vi "Periodic Tasks.vi"(0 "error in":errorcluster) -> ()   [LabVIEW 2020]
doc: "All TeleOperated, Autonomous, and Test controller logic are located here. Sensor reads and actuator commands are run inside of parallel loops. Most FRC 4265 code should be placed here."
uses:
  dsdata.vi
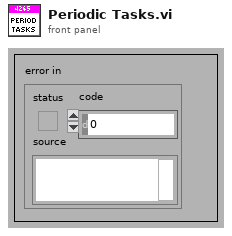
[diagram p1: front panel]
types:
  T1 = typedef "WPI_DriverStationRobotMode2.ctl" = enum16{"Autonomous Disabled", "Autonomous Enabled", "Teleop Disabled", "Teleop Enabled", "Disconnected", "Finish", "Test Disabled", "Test Enabled", "Emergency Stopped"}
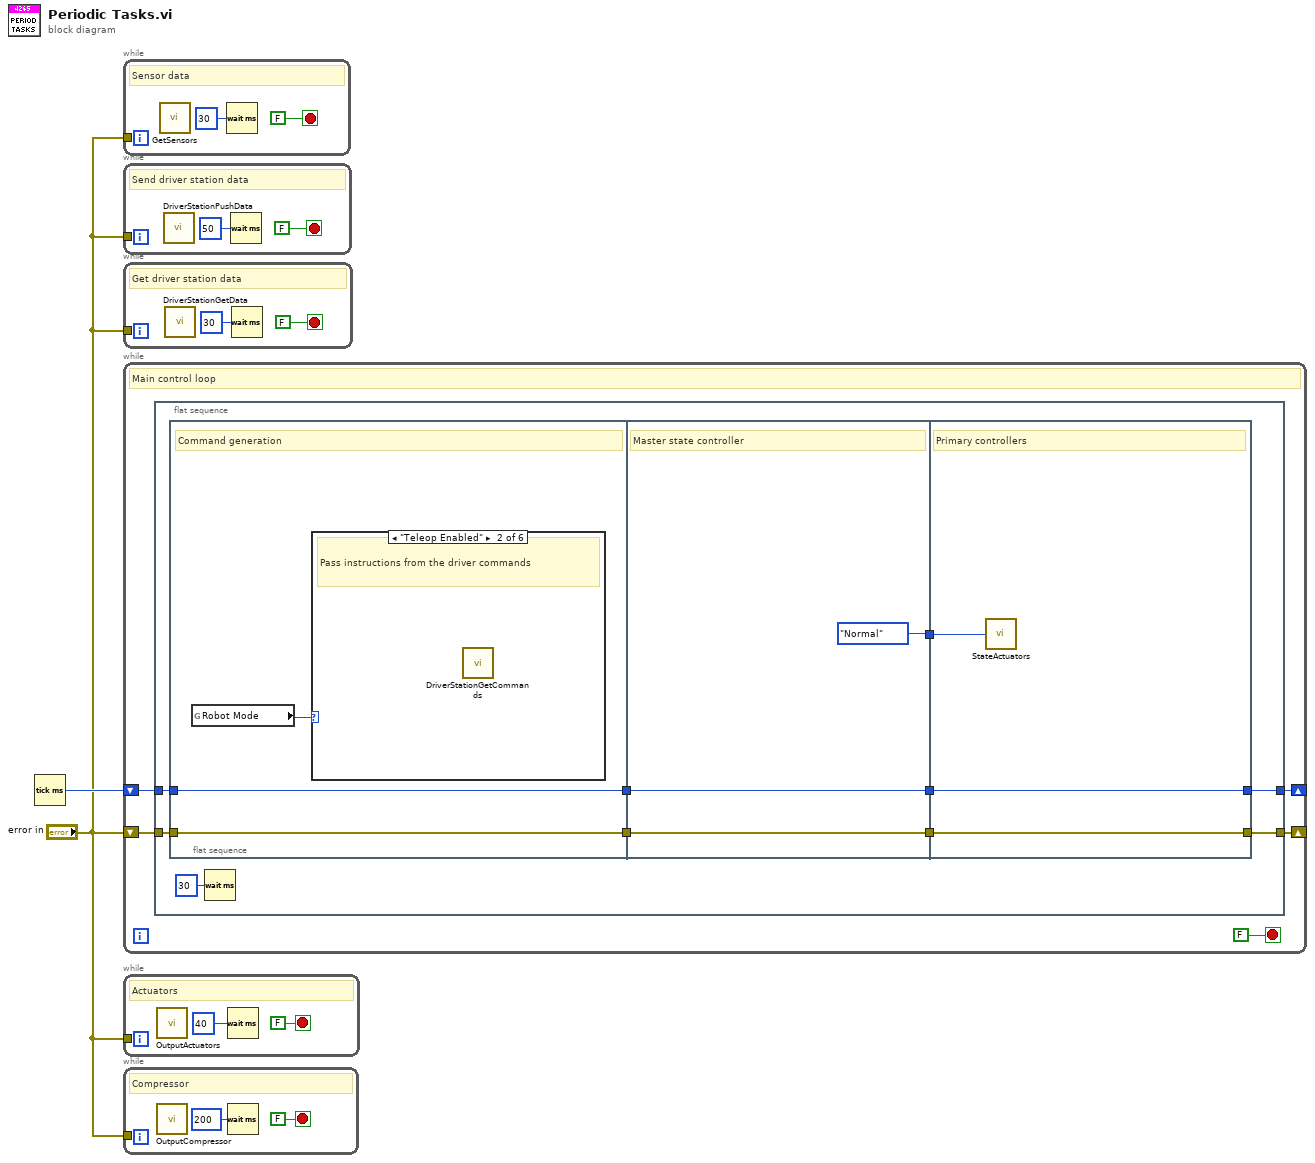
[diagram p0: block diagram]
diagram:
  n1 = Tick Count (ms)() -> (millisecond timer value=w2:u32)
  n2 = while {
    tunnel: "error in" -> [_]
    stop <- FALSE stop-if-true
    # "Sensor data"
    n3 = call "GetSensors.vi"() -> ()  [unwired: 1 in]
    n4 = Wait (ms)(milliseconds to wait=u32 30) -> ()  [unwired: 1 out]
  }
  n5 = while {
    tunnel: "error in" -> [_]
    stop <- FALSE stop-if-true
    # "Send driver station data"
    n6 = call "DriverStationPushData.vi"() -> ()  [unwired: 1 in]
    n7 = Wait (ms)(milliseconds to wait=u32 50) -> ()  [unwired: 1 out]
  }
  n8 = while {
    tunnel: "error in" -> [_]
    stop <- FALSE stop-if-true
    # "Get driver station data"
    n9 = call "DriverStationGetData.vi"() -> ()  [unwired: 1 in]
    n10 = Wait (ms)(milliseconds to wait=u32 30) -> ()  [unwired: 1 out]
  }
  n11 = while {
    shift-right: [w9] -> _
    shift-left: w2 -> [w10]
    shift-right: [w11] -> _
    shift-left: "error in" -> [w12]
    stop <- FALSE stop-if-true
    # "Main control loop"
    n12 = flat-sequence {
      tunnel: [w22] -> w9
      tunnel: [w23] -> w11
      tunnel: w10 -> [w15]
      tunnel: w12 -> [w16]
      frame #0 {
        n13 = flat-sequence {
          tunnel: [w26] -> w21
          tunnel: w16 -> [w26]
          tunnel: [w25] -> w20
          tunnel: w15 -> [w25]
          tunnel: [enum16{"Normal"}."Normal"] -> w17
          tunnel: w21 -> [w29]
          tunnel: [w29] -> w18
          tunnel: w20 -> [w28]
          tunnel: [w28] -> w19
          tunnel: [w32] -> w23
          tunnel: [w31] -> w22
          tunnel: w19 -> [w31]
          tunnel: w18 -> [w32]
          tunnel: w17 -> [w30]
          frame #0 {
            # "Command generation"
            n14 = global read "dsdata.vi" "Robot Mode"() -> (w24:T1)
            n15 = case shown="\"Teleop Enabled\"" w24 {
              frame "Autonomous Disabled".."Teleop Disabled", Default {
                # "Robot is disabled, super test mode is available"
              }
              frame "Teleop Enabled" {
                # "Pass instructions from the driver commands"
                n16 = call "DriverStationGetCommands.vi"() -> ()  [unwired: 12 in]
              }
              frame "Finish" {
                # "Clean up operations are in the Finish.vi in RobotMain.vi"
              }
              frame "Test Disabled", "Test Enabled" {
                # "Use TestActuatorInterlock.vi for implimenting test code"
              }
              frame "Disconnected" {
                # "Communications have failed"
              }
              frame "Emergency Stopped" {
                # "Robot has been emergency stopped"
              }
            }
          }
          frame #1 {
            # "Master state controller"
          }
          frame #2 {
            # "Primary controllers"
            n17 = call "StateActuators.vi"("Master State"=w30) -> ()
          }
        }
        n18 = Wait (ms)(milliseconds to wait=u32 30) -> ()  [unwired: 1 out]
      }
    }
  }
  n19 = while {
    tunnel: "error in" -> [_]
    stop <- FALSE stop-if-true
    # "Actuators"
    n20 = call "OutputActuators.vi"() -> ()  [unwired: 1 in]
    n21 = Wait (ms)(milliseconds to wait=u32 40) -> ()  [unwired: 1 out]
  }
  n22 = while {
    tunnel: "error in" -> [_]
    stop <- FALSE stop-if-true
    # "Compressor"
    n23 = call "OutputCompressor.vi"() -> ()  [unwired: 1 in]
    n24 = Wait (ms)(milliseconds to wait=u32 200) -> ()  [unwired: 1 out]
  }
